vi "Write Subpanel Refnum.vi"(7 "Force Overwrite? (F)":bool, 8 "error in (no error)":errorcluster, 10 "SubPnl Refnum":refnum<vi>, 11 "IController In":refnum<class "IController.lvclass">) -> (0 "error out":errorcluster, 3 "IController Out":refnum<class "IController.lvclass">)   [LabVIEW 2015, in "IController.lvlib" / "IController.lvclass"]
uses:
  IController.lvclass
  IController.lvclass/IController.ctl
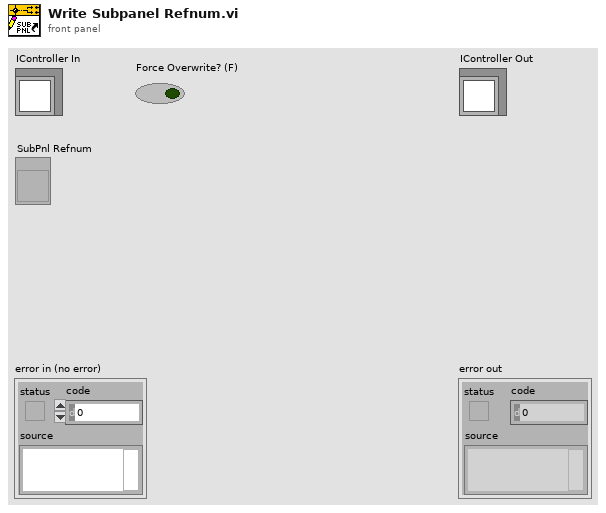
[diagram p1: front panel]
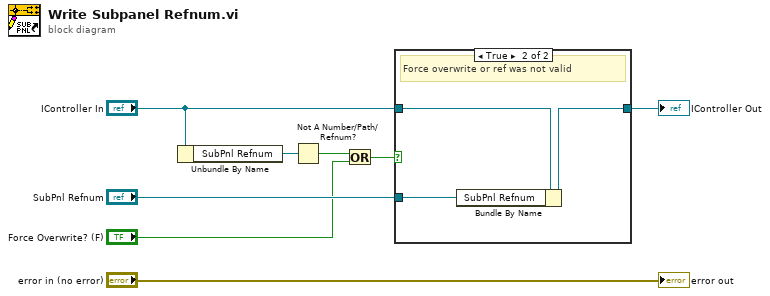
[diagram p0: block diagram]
diagram:
  n1 = Unbundle By Name("IController In") -> ("SubPnl Refnum"=w5:refnum<vi>)
  n2 = Not A Number/Path/Refnum?(number/path/refnum=w5) -> (NaN/Path/Refnum?=w4:bool)
  n3 = Or(x=w4, y="Force Overwrite? (F)") -> (x .or. y?=w1:bool)
  n4 = case shown="True" w1 {
    tunnel: [w9 w12] -> w7
    tunnel: "SubPnl Refnum" -> [_ w11]
    tunnel: "IController In" -> [w9 w10]
    frame False {
      # "Keep pre-existing refnum"
    }
    frame True {
      # "Force overwrite or ref was not valid"
      n5 = Bundle By Name(cluster=w10, "SubPnl Refnum"=w11) -> (w12:refnum<class "IController.lvclass">)
    }
  }
  "IController Out" <- w7
  "error out" <- "error in (no error)"
